vi "CSV_Setup_Data_Append.vi"(8 "input cluster":T2={"Pinch-valve"="Test Sample", "XLP 6000 Pump"="MRJ", "Camera1"="", "Camera2"="", "Img_Capt"=FALSE, "Actuator"=FALSE, "Pump"=FALSE, "Cam 1"=FALSE, "Cam 2"=FALSE, "Empty_Refill"=FALSE, "Crop"=FALSE, "Light intensity"=0, "Exposure Time"=0.0, "Sample Name"="", "Operator"="", "Calibration 1"=path "C:/Users/au540322/Desktop/IHS_Project/images/Debris/Debris_0/Debris_0_2019_06_01-23-32-49-686.PNG", "Calibration 2"=path "C:/Users/au540322/Desktop/IHS_Project/images/Debris/Debris_0/Debris_0_2019_06_01-23-32-49-686.PNG", "Framerate"=1, "Timeout Sample"=1, "Collection date"="", "Sample size threshold"=10, "Empty start"=1, "Command"="", "Station"="", "Species Name"="", "Other Notes"="", "Aperture"=enum."Item 3", "Image Process Queue Size"=100, "Image Save Queue Size"=0, "Overload threshold"=0, "Max Framerate"=0, "Rectangle 1"={"Left"=0, "Top"=0, "Right"=0, "Bottom"=0, "Rotation"=0.0}, "Rectangle 2"={"Left"=0, "Top"=100, "Right"=100, "Bottom"=0, "Rotation"=0.0}, "Detection Region %"=200.0, "Detect 1"=path "C:/Users/au540322/Desktop/IHS_Project/images/Debris/Debris_0/Debris_0_2019_06_01-23-32-49-686.PNG", "Detect 2"=path "C:/Users/au540322/Desktop/IHS_Project/images/Debris/Debris_0/Debris_0_2019_06_01-23-32-49-686.PNG", "Max large object threshold"=500, "Open(T)/Close(F)"=FALSE, "Img_Capt Begin"=FALSE, "Dispense Speed"=0, "Flush Size"=0, "Location"="", "Latitude"="", "Longitude"="", "Determiner"="", "Sex"="", "Camera1_Img"=refnum, "Camera2_Img"=refnum, "Img1_Orig_Disp"=refnum, "Img2_Orig_Disp"=refnum, "Img1_Orig_RGB"=refnum, "Img2_Orig_RGB"=refnum, "Blue_Plane_Extract"=refnum, "Subtracted_Plane"=refnum, "Img1_Binary"=refnum, "Img2_Binary"=refnum, "Crop_Mask"=refnum, "Img1_Save"=refnum, "Img2_Save"=refnum, "Img1_Cali_Full"=refnum, "Img2_Cali_Full"=refnum, "Img1_Cali_Detect"=refnum, "Img2_Cali_Detect"=refnum, "Cam 1 queue"=refnum, "Cam 2 queue"=refnum, "Cam 1 - save queue"=refnum, "Cam 2 - save queue"=refnum, "Overlay_Ring"=0, "SystemVersion"=0, "System Serial"="", "Legacy Cam Attributes"=FALSE, "Camera Orientation 1"="", "Camera Orientation 2"="", "Pixel to mm 1"=0.0, "Pixel to mm 2"=0.0, "CAM1 Model"=enum."a2A5328-15ucBAS", "CAM2 Model"=enum."a2A5328-15ucBAS", "Flush Insect"=FALSE, "Pump Size"=FALSE, "Barcode"="", "Phase3"=FALSE, "Mega F3"="", "Container nr."=0.0, "Flush Error"=TRUE} {"SystemVersion" items=["Standard", "XL"]; "Overlay_Ring" items=["Session Data", "Extended Setup", "Buffer", "Camera", "Dispenser", "Stats", "Connections"]; "Flush Size" min=1; "Dispense Speed" min=1; "Rectangle 2"."Rotation" format="%.2f"; "Rectangle 2"."Left" scale=0.0..1024.0; "Rectangle 2"."Right" scale=0.0..1024.0; "Rectangle 1"."Rotation" format="%.2f"; "Rectangle 1"."Left" scale=0.0..1024.0; "Rectangle 1"."Right" scale=0.0..1024.0; "Max Framerate" min=1; "Overload threshold" min=1; "Image Save Queue Size" min=1; "Image Process Queue Size" min=1; "Empty start" min=1; "Sample size threshold" min=1; "Framerate" min=1; "Light intensity" scale=0.0..100.0}, 9 "Sample cluster":T1, 10 "Sample Name":string, 11 "Image path":string) -> (2 "File Path":string, 3 "Sample Name dup":string)   [LabVIEW 2024]
uses:
  controls/Data.ctl
  <vilib>/userDefined/High Color/IMAQdx.ctl
  <vilib>/vision/Image Controls.llb/IMAQ Image.ctl
  <vilib>/Utility/file.llb/Write Delimited Spreadsheet (string).vi
panel:
  out "string":string
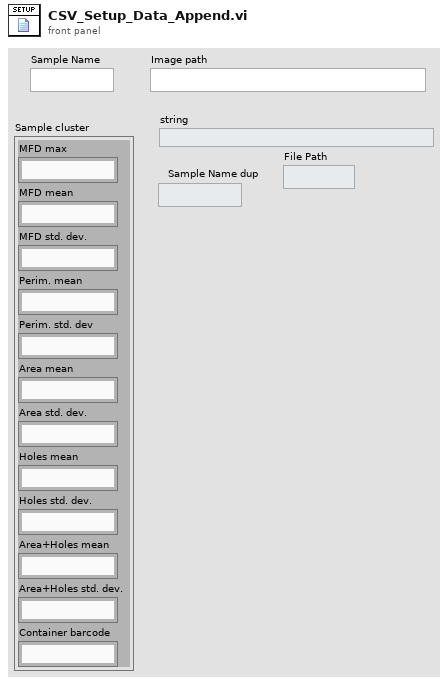
[diagram p1: front panel]
types:
  T1 = cluster{"MFD max":string, "MFD mean":string, "MFD std. dev.":string, "Perim. mean":string, "Perim. std. dev":string, "Area mean":string, "Area std. dev.":string, "Holes mean":string, "Holes std. dev.":string, "Area+Holes mean":string, "Area+Holes std. dev.":string, "Container barcode":string}
  T2 = typedef "Data.ctl" = cluster{"Pinch-valve":refnum<visa-resource-name>, "XLP 6000 Pump":refnum<visa-resource-name>, "Camera1":T3, "Camera2":T3, "Img_Capt":bool, "Actuator":bool, "Pump":bool, "Cam 1":bool, "Cam 2":bool, "Empty_Refill":bool, "Crop":bool, "Light intensity":i32, "Exposure Time":dbl, "Sample Name":string, "Operator":string, "Calibration 1":path, "Calibration 2":path, "Framerate":i32, "Timeout Sample":i32, "Collection date":string, "Sample size threshold":i32, "Empty start":u32, "Command":string, "Station":string, "Species Name":string, "Other Notes":string, "Aperture":enum32{"Item 0", "Item 1", "Item 2", "Item 3"}, "Image Process Queue Size":i32, "Image Save Queue Size":i32, "Overload threshold":i32, "Max Framerate":i32, "Rectangle 1":T4, "Rectangle 2":T4, "Detection Region %":dbl, "Detect 1":path, "Detect 2":path, "Max large object threshold":i32, "Open(T)/Close(F)":bool, "Img_Capt Begin":bool, "Dispense Speed":i32, "Flush Size":i32, "Location":string, "Latitude":string, "Longitude":string, "Determiner":string, "Sex":string, "Camera1_Img":T5, "Camera2_Img":T5, "Img1_Orig_Disp":T5, "Img2_Orig_Disp":T5, "Img1_Orig_RGB":T5, "Img2_Orig_RGB":T5, "Blue_Plane_Extract":T5, "Subtracted_Plane":T5, "Img1_Binary":T5, "Img2_Binary":T5, "Crop_Mask":T5, "Img1_Save":T5, "Img2_Save":T5, "Img1_Cali_Full":T5, "Img2_Cali_Full":T5, "Img1_Cali_Detect":T5, "Img2_Cali_Detect":T5, "Cam 1 queue":refnum<queue>, "Cam 2 queue":refnum<queue>, "Cam 1 - save queue":refnum<queue>, "Cam 2 - save queue":refnum<queue>, "Overlay_Ring":u16, "SystemVersion":u16, "System Serial":string, "Legacy Cam Attributes":bool, "Camera Orientation 1":string, "Camera Orientation 2":string, "Pixel to mm 1":dbl, "Pixel to mm 2":dbl, "CAM1 Model":enum16{"a2A5328-15ucBAS", "acA1920-155uc"}, "CAM2 Model":enum16{"a2A5328-15ucBAS", "acA1920-155uc"}, "Flush Insect":bool, "Pump Size":bool, "Barcode":string, "Phase3":bool, "Mega F3":refnum<visa-resource-name>, "Container nr.":dbl, "Flush Error":bool}
  T3 = typedef "IMAQdx.ctl" = refnum<k21>
  T4 = typedef "IMAQ Rectangle" = cluster{"Left":i32, "Top":i32, "Right":i32, "Bottom":i32, "Rotation":dbl}
  T5 = typedef "IMAQ Image.ctl" = refnum<image>
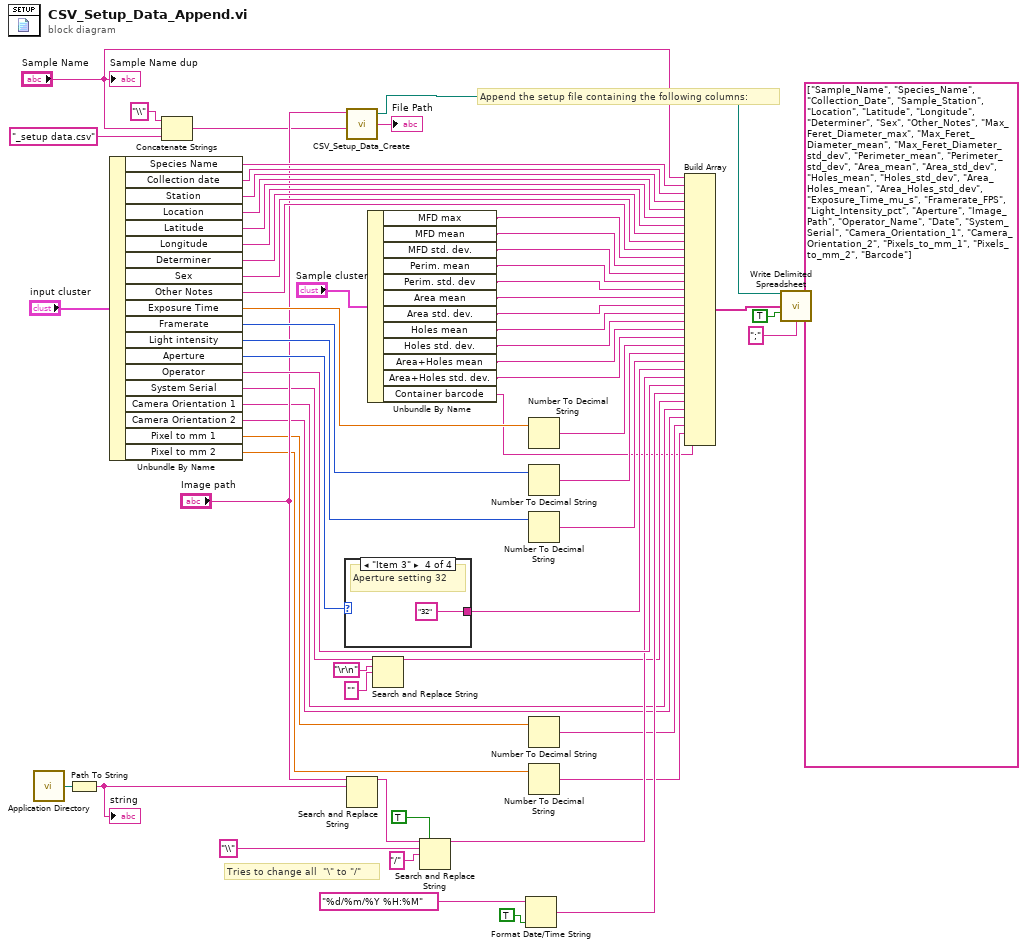
[diagram p0: block diagram]
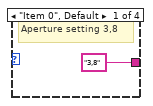
[diagram p2: hidden frame]
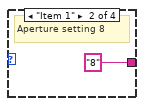
[diagram p3: hidden frame]
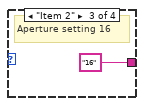
[diagram p4: hidden frame]
diagram:
  (unwired) string[] ["Sample_Name", "Species_Name", "Collection_Date", "Sample_Station", "Location", "Latitude", "Longitude", "Determiner", "Sex", "Other_Notes", "Max_Feret_Diameter_max", "Max_Feret_Diameter_mean", "Max_Feret_Diameter_std_dev", "Perimeter_mean", "Perimeter_std_dev", "Area_mean", "Area_std_dev", "Holes_mean", "Holes_std_dev", "Area_Holes_mean", "Area_Holes_std_dev", "Exposure_Time_mu_s", "Framerate_FPS", "Light_Intensity_pct", "Aperture", "Image_Path", "Operator_Name", "Date", "System_Serial", "Camera_Orientation_1", "Camera_Orientation_2", "Pixels_to_mm_1", "Pixels_to_mm_2", "Barcode"]
  # "Tries to change all  \"\\\" to \"/\""
  # "Append the setup file containing the following columns:"
  n1 = call <vilib>:"Application Directory.vi"() -> ("Application Directory"=w59:path)
  n2 = Path To String(path=w59) -> (string=w58:string)
  "string" <- w58
  n3 = Unbundle By Name("input cluster") -> ("Species Name"=w39:string, "Collection date"=w40:string, "Station"=w41:string, "Location"=w42:string, "Latitude"=w43:string, "Longitude"=w44:string, "Determiner"=w45:string, "Sex"=w46:string, "Other Notes"=w47:string, "Exposure Time"=w57:dbl, "Framerate"=w56:i32, "Light intensity"=w55:i32, "Aperture"=w54:enum32{"Item 0", "Item 1", "Item 2", "Item 3"}, "Operator"=w49:string, "System Serial"=w18:string, "Camera Orientation 1"=w24:string, "Camera Orientation 2"=w23:string, "Pixel to mm 1"=w22:dbl, "Pixel to mm 2"=w20:dbl)
  n4 = Concatenate Strings("\\" ("string"), "Sample Name", "_setup data.csv") -> (w32:string)
  n5 = case shown="\"Item 3\"" w54 {
    tunnel: ["3,8" "8" "16" "32"] -> w50
    frame "Item 0", Default {
      # "Aperture setting 3,8"
    }
    frame "Item 1" {
      # "Aperture setting 8"
    }
    frame "Item 2" {
      # "Aperture setting 16"
    }
    frame "Item 3" {
      # "Aperture setting 32"
    }
  }
  n6 = call "CSV_Setup_Data_Create.vi"("Setup Data File"=w32, "Setup Data path"="Image path") -> ("File Path"=→"File Path":string, "Setup Data File path"=w34:path)  [unwired: 2 in, 1 out]
  n7 = Search and Replace String(input string="Image path", search string=w58) -> (result string=w26:string)  [unwired: 6 in, 3 out]
  n8 = Unbundle By Name("Sample cluster") -> ("MFD max"=w12:string, "MFD mean"=w11:string, "MFD std. dev."=w10:string, "Perim. mean"=w9:string, "Perim. std. dev"=w8:string, "Area mean"=w7:string, "Area std. dev."=w6:string, "Holes mean"=w5:string, "Holes std. dev."=w4:string, "Area+Holes mean"=w3:string, "Area+Holes std. dev."=w2:string, "Container barcode"=w1:string)
  n9 = Search and Replace String(input string=w18, search string="\r\n", replace string="" ("replace string (\"\")")) -> (result string=w17:string)  [unwired: 5 in, 3 out]
  n10 = Search and Replace String(replace all?=TRUE ("replace all? (F)"), input string=w26, search string="\\", replace string="/" ("replace string (\"\")")) -> (result string=w25:string)  [unwired: 4 in, 3 out]
  n11 = Format Date/Time String(time format string (%c)="%d/%m/%Y %H:%M", UTC format=TRUE) -> (date/time string=w48:string)  [unwired: 1 in]
  n12 = Number To Decimal String(number=w57) -> (decimal integer string=w53:string)  [unwired: 1 in]
  n13 = Number To Decimal String(number=w56) -> (decimal integer string=w52:string)  [unwired: 1 in]
  n14 = Number To Decimal String(number=w55) -> (decimal integer string=w51:string)  [unwired: 1 in]
  n15 = Number To Decimal String(number=w22) -> (decimal integer string=w21:string)  [unwired: 1 in]
  n16 = Number To Decimal String(number=w20) -> (decimal integer string=w19:string)  [unwired: 1 in]
  n17 = Build Array("Sample Name", w39, w40, w41, w42, w43, w44, w45, w46, w47, w12, w11, w10, w9, w8, w7, w6, w5, w4, w3, w2, w53, w52, w51, w50, w25, w49, w48, w17, w24, w23, w21, w19, w1) -> (w14:string[])
  n18 = call-poly <vilib>:"Write Delimited Spreadsheet.vi"("file path (dialog if empty)"=w34, "1D data"=w14, "append to file? (new file:F)"=TRUE, "delimiter (\\t)"=";" ("delimiter (\\t)")) -> ()  [unwired: 10 in, 2 out]
  "Sample Name dup" <- "Sample Name"
